vi "ABB Report entered data.vi"(9 "result string in":string, 10 "Efficiency Units":u16(ring) items=["METRIC", "IMPERIAL", "", "", ""], 11 "Efficiency Standard":u16(ring) items=["IEC", "NEMA"]) -> (1 "result string out":string)   [LabVIEW 2017]
uses:
  ABB global.vi
panel:
  out "loads":string[](array[string])
  out "PF&Effy":string[](array[string])
  out "# entries":string[](array[string])
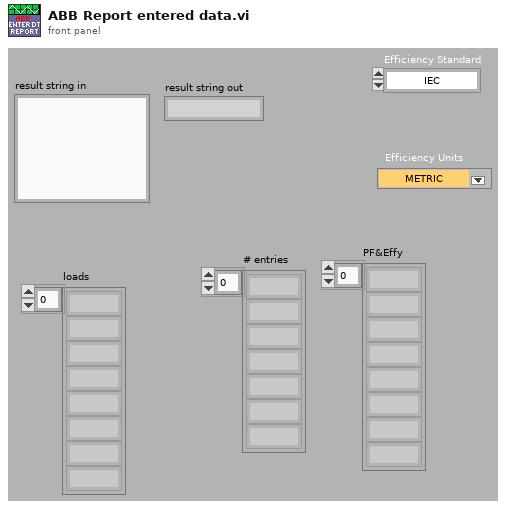
[diagram p1: front panel]
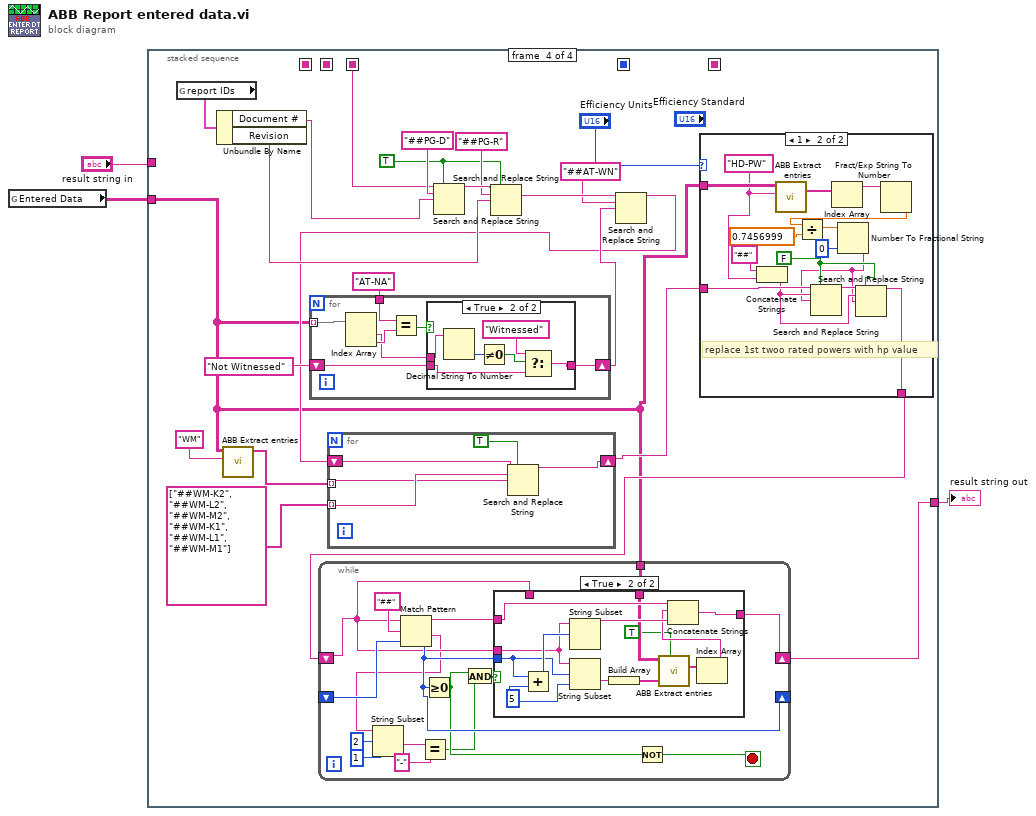
[diagram p0: block diagram]
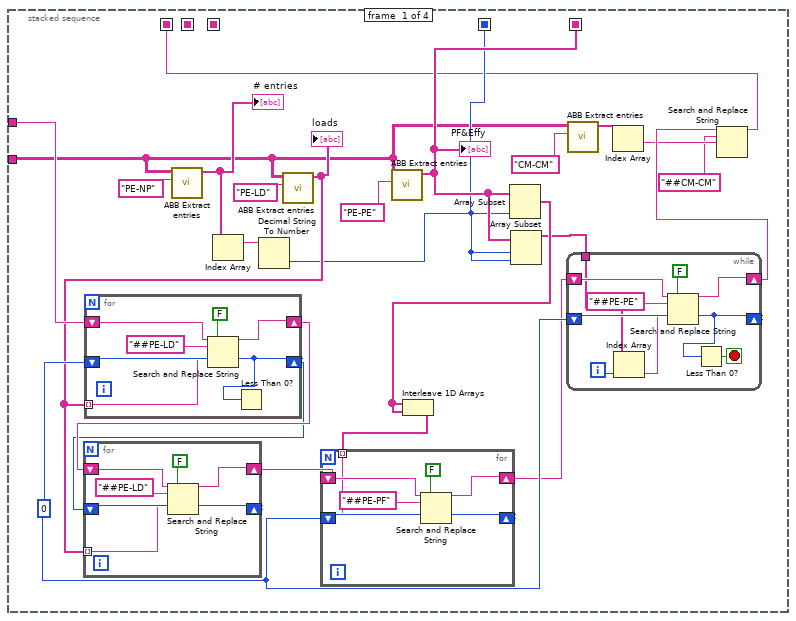
[diagram p2: hidden frame]
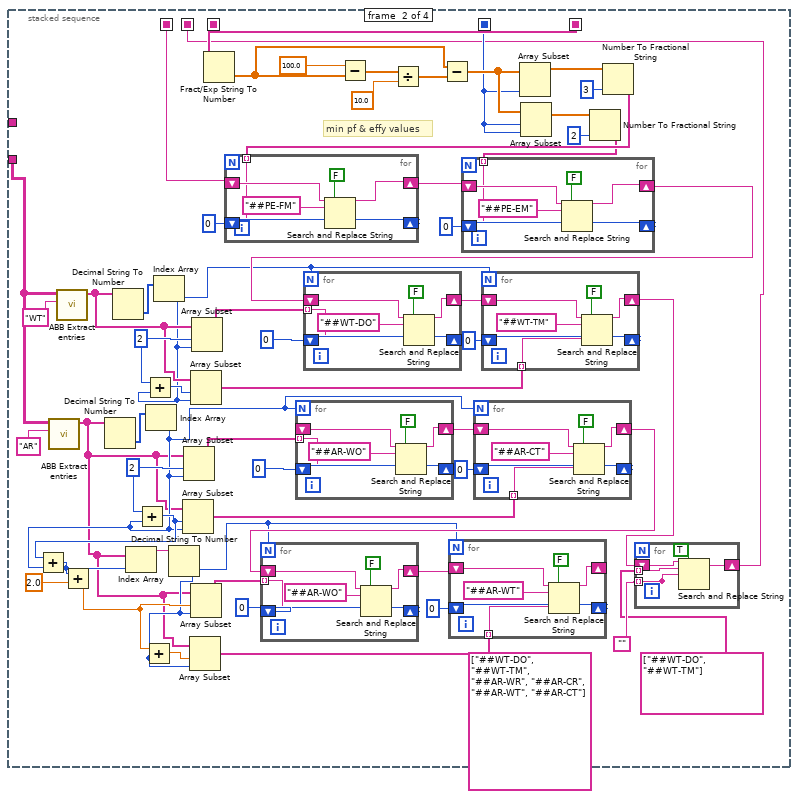
[diagram p3: hidden frame]
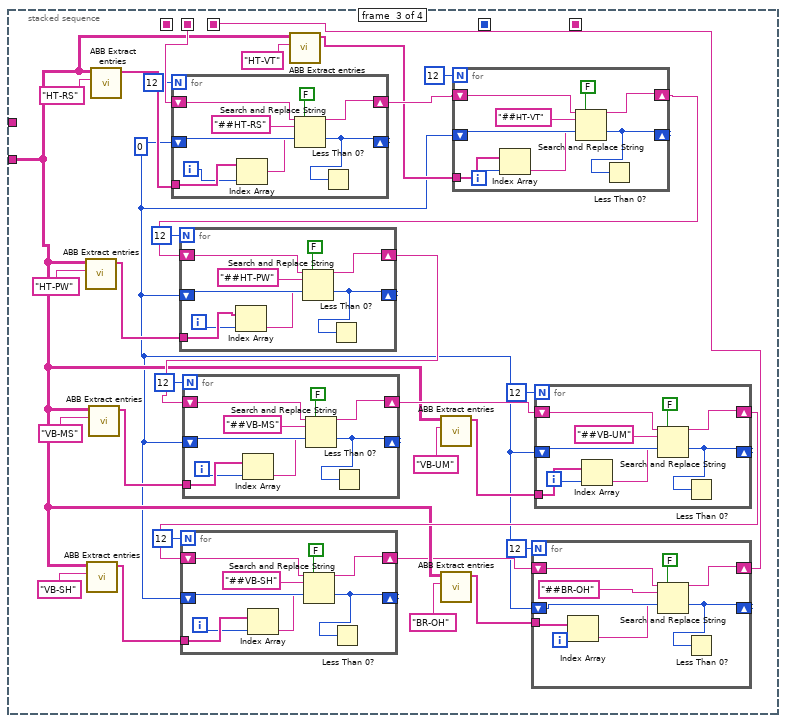
[diagram p4: hidden frame]
diagram:
  n1 = global read "ABB global.vi" "Entered Data"() -> (w1:string[][])
  n2 = stacked-sequence {
    seq-local: [w7 _ _ _] -> [_ w105 _ _]
    seq-local: [w12 _ _ _] -> [_ w116 _ _]
    seq-local: [w11 _ _ _] -> [_ w109 _ _]
    seq-local: [_ w61 _ _] -> [_ _ w206 _]
    seq-local: [_ _ w187 _] -> [_ _ _ w281]
    tunnel: [_ _ _ w280] -> w3
    tunnel: "result string in" -> [w20 _ _ _]
    tunnel: w1 -> [w9 w80 w189 w273]
    frame #0 {
      w21 = 0 ("offset past replacement")
      n3 = call "ABB Extract entries.vi"("Entry ID"="PE-NP" ("element"), "Entry table in"=w9) -> ("Selected Entries"=w24:string[])  [unwired: 9 in]
      "# entries" <- w24
      n4 = Index Array(array=w24) -> (element=w23:string)  [unwired: 1 in]
      n5 = Decimal String To Number(string=w23) -> (number=w11:i32)  [unwired: 2 in, 1 out]
      n6 = call "ABB Extract entries.vi"("Entry ID"="PE-LD" ("element"), "Entry table in"=w9) -> ("Selected Entries"=w17:string[])  [unwired: 9 in]
      "loads" <- w17
      n7 = for {
        shift-right: [w46] -> w19
        shift-left: w20 -> [w48]
        tunnel: w17 -> [w42] mode=indexing
        shift-right: [w43] -> w18
        shift-left: w21 -> [w45]
        n8 = Search and Replace String(replace all?=FALSE ("replace all? (F)"), input string=w48, search string="##PE-LD", replace string=w42, offset=w45) -> (result string=w46:string, offset past replacement=w43:i32)  [unwired: 3 in, 2 out]
        n9 = Less Than 0?(x=w43) -> ()  [unwired: 1 out]
      }
      n10 = for {
        shift-right: [w39] -> w22
        shift-left: w19 -> [w41]
        tunnel: w17 -> [w35] mode=indexing
        shift-right: [w36] -> _
        shift-left: w18 -> [w38]
        n11 = Search and Replace String(replace all?=FALSE ("replace all? (F)"), input string=w41, search string="##PE-LD", replace string=w35, offset=w38) -> (result string=w39:string, offset past replacement=w36:i32)  [unwired: 3 in, 2 out]
      }
      n12 = call "ABB Extract entries.vi"("Entry ID"="PE-PE", "Entry table in"=w9) -> ("Selected Entries"=w12:string[])  [unwired: 9 in]
      "PF&Effy" <- w12
      n13 = Array Subset(array=w12, length=w11) -> (w14:string[])  [unwired: 1 in]
      n14 = Interleave 1D Arrays(w14, w14) -> (w15:string[])
      n15 = for {
        shift-right: [w32] -> w16
        shift-left: w22 -> [w34]
        shift-right: [w29] -> _
        shift-left: w21 -> [w31]
        tunnel: w15 -> [w28] mode=indexing
        n16 = Search and Replace String(replace all?=FALSE ("replace all? (F)"), input string=w34, search string="##PE-PF", replace string=w28, offset=w31) -> (result string=w32:string, offset past replacement=w29:i32)  [unwired: 3 in, 2 out]
      }
      n17 = Array Subset(array=w12, index=w11, length=w11) -> (w13:string[])
      n18 = while {
        shift-right: [w56] -> w6
        shift-left: w16 -> [w58]
        shift-right: [w52] -> _
        shift-left: w21 -> [w55]
        tunnel: w13 -> [w49]
        i -> [w51]
        stop <- w53 stop-if-true
        n19 = Index Array(array=w49, index=w51) -> (element=w50:string)
        n20 = Search and Replace String(replace all?=FALSE ("replace all? (F)"), input string=w58, search string="##PE-PE", replace string=w50, offset=w55) -> (result string=w56:string, offset past replacement=w52:i32)  [unwired: 3 in, 2 out]
        n21 = Less Than 0?(x=w52) -> (x < 0?=w53:bool)
      }
      n22 = call "ABB Extract entries.vi"("Entry ID"="CM-CM", "Entry table in"=w9) -> ("Selected Entries"=w8:string[])  [unwired: 9 in]
      n23 = Index Array(array=w8) -> (element=w5:string)  [unwired: 1 in]
      n24 = Search and Replace String(input string=w6, search string="##CM-CM", replace string=w5) -> (result string=w7:string)  [unwired: 5 in, 3 out]
    }
    frame #1 {
      (unwired) string[] ["##WT-DO", "##WT-TM", "##AR-WR", "##AR-CR", "##AR-WT", "##AR-CT"]
      w84 = 2 ("index")
      w93 = 2 ("index")
      # "min pf & effy values"
      n25 = call "ABB Extract entries.vi"("Entry ID"="AR", "Entry table in"=w80) -> ("Selected Entries"=w63:string[])  [unwired: 9 in]
      n26 = call "ABB Extract entries.vi"("Entry ID"="WT", "Entry table in"=w80) -> ("Selected Entries"=w89:string[])  [unwired: 9 in]
      n27 = Decimal String To Number(string=w63) -> (number=w82:i32[])  [unwired: 2 in, 1 out]
      n28 = Decimal String To Number(string=w89) -> (number=w95:i32[])  [unwired: 2 in, 1 out]
      n29 = Index Array(array=w82) -> (element=w66:i32)  [unwired: 1 in]
      n30 = Add(x=w84, y=w66) -> (x+y=w71:i32)
      n31 = Add(x=w71, y=w66) -> (x+y=w70:i32)
      n32 = Add(x=w70, y=2.0) -> (x+y=w68:dbl)
      n33 = Index Array(array=w63, index=w70) -> (element=w67:string)
      n34 = Index Array(array=w95) -> (element=w64:i32)  [unwired: 1 in]
      n35 = Add(x=w93, y=w64) -> (x+y=w92:i32)
      n36 = Decimal String To Number(string=w67) -> (number=w65:i32)  [unwired: 2 in, 1 out]
      n37 = Add(x=w68, y=w65) -> (x+y=w76:dbl)
      n38 = Array Subset(array=w63, index=w71, length=w66) -> (w87:string[])
      n39 = Array Subset(array=w63, index=w84, length=w66) -> (w83:string[])
      n40 = Array Subset(array=w63, index=w76, length=w65) -> (w73:string[])
      n41 = Array Subset(array=w89, index=w92, length=w64) -> (w88:string[])
      n42 = Array Subset(array=w63, index=w68, length=w65) -> (w77:string[])
      n43 = Array Subset(array=w89, index=w93, length=w64) -> (w94:string[])
      n44 = Fract/Exp String To Number(string=w116) -> (number=w112:dbl[])  [unwired: 3 in, 1 out]
      n45 = for {
        N: w66 -> [_]
        shift-right: [w147] -> w85
        shift-left: _ -> [w149]
        shift-right: [w144] -> _
        shift-left: 0 ("offset past replacement") -> [w146]
        tunnel: w83 -> [w143] mode=indexing
        n46 = Search and Replace String(replace all?=FALSE ("replace all? (F)"), input string=w149, search string="##AR-WO", replace string=w143, offset=w146) -> (result string=w147:string, offset past replacement=w144:i32)  [unwired: 3 in, 2 out]
      }
      n47 = Subtract(x=100.0, y=w112) -> (x-y=w114:dbl[])
      n48 = Divide(x=w114, y=10.0) -> (x/y=w111:dbl[])
      n49 = Subtract(x=w112, y=w111) -> (x-y=w110:dbl[])
      n50 = for {
        N: w66 -> [_]
        shift-right: [w140] -> w72
        shift-left: w85 -> [w142]
        shift-right: [w137] -> _
        shift-left: 0 ("offset past replacement") -> [w139]
        tunnel: w87 -> [w136] mode=indexing
        n51 = Search and Replace String(replace all?=FALSE ("replace all? (F)"), input string=w142, search string="##AR-CT", replace string=w136, offset=w139) -> (result string=w140:string, offset past replacement=w137:i32)  [unwired: 3 in, 2 out]
      }
      n52 = for {
        N: w65 -> [_]
        shift-right: [w133] -> w75
        shift-left: w72 -> [w135]
        shift-right: [w130] -> _
        shift-left: 0 ("offset past replacement") -> [w132]
        tunnel: w77 -> [w129] mode=indexing
        n53 = Search and Replace String(replace all?=FALSE ("replace all? (F)"), input string=w135, search string="##AR-WO", replace string=w129, offset=w132) -> (result string=w133:string, offset past replacement=w130:i32)  [unwired: 3 in, 2 out]
      }
      n54 = for {
        N: w65 -> [_]
        shift-right: [w126] -> _
        shift-left: w75 -> [w128]
        shift-right: [w123] -> _
        shift-left: 0 ("offset past replacement") -> [w125]
        tunnel: w73 -> [w122] mode=indexing
        n55 = Search and Replace String(replace all?=FALSE ("replace all? (F)"), input string=w128, search string="##AR-WT", replace string=w122, offset=w125) -> (result string=w126:string, offset past replacement=w123:i32)  [unwired: 3 in, 2 out]
      }
      n56 = Array Subset(array=w110, length=w109) -> (w108:dbl[])  [unwired: 1 in]
      n57 = Array Subset(array=w110, index=w109, length=w109) -> (w102:dbl[])
      n58 = Number To Fractional String(number=w102, precision (6)=i16 2) -> (F-format string=w100:string[])  [unwired: 2 in]
      n59 = Number To Fractional String(number=w108, precision (6)=i16 3) -> (F-format string=w106:string[])  [unwired: 2 in]
      n60 = for {
        shift-right: [w175] -> w103
        shift-left: w105 -> [w177]
        shift-right: [w172] -> _
        shift-left: 0 ("offset past replacement") -> [w174]
        tunnel: w106 -> [w171] mode=indexing
        n61 = Search and Replace String(replace all?=FALSE ("replace all? (F)"), input string=w177, search string="##PE-FM", replace string=w171, offset=w174) -> (result string=w175:string, offset past replacement=w172:i32)  [unwired: 3 in, 2 out]
      }
      n62 = for {
        shift-right: [w168] -> w98
        shift-left: w103 -> [w170]
        shift-right: [w165] -> _
        shift-left: 0 ("offset past replacement") -> [w167]
        tunnel: w100 -> [w164] mode=indexing
        n63 = Search and Replace String(replace all?=FALSE ("replace all? (F)"), input string=w170, search string="##PE-EM", replace string=w164, offset=w167) -> (result string=w168:string, offset past replacement=w165:i32)  [unwired: 3 in, 2 out]
      }
      n64 = for {
        N: w64 -> [_]
        shift-right: [w161] -> w91
        shift-left: w98 -> [w163]
        shift-right: [w158] -> _
        shift-left: 0 ("offset past replacement") -> [w160]
        tunnel: w94 -> [w157] mode=indexing
        n65 = Search and Replace String(replace all?=FALSE ("replace all? (F)"), input string=w163, search string="##WT-DO", replace string=w157, offset=w160) -> (result string=w161:string, offset past replacement=w158:i32)  [unwired: 3 in, 2 out]
      }
      n66 = for {
        N: w64 -> [_]
        shift-right: [w154] -> w60
        shift-left: w91 -> [w156]
        shift-right: [w151] -> _
        shift-left: 0 ("offset past replacement") -> [w153]
        tunnel: w88 -> [w150] mode=indexing
        n67 = Search and Replace String(replace all?=FALSE ("replace all? (F)"), input string=w156, search string="##WT-TM", replace string=w150, offset=w153) -> (result string=w154:string, offset past replacement=w151:i32)  [unwired: 3 in, 2 out]
      }
      n68 = for {
        shift-right: [w120] -> w61
        shift-left: w60 -> [w121]
        tunnel: string[] ["##WT-DO", "##WT-TM"] -> [w118] mode=indexing
        tunnel: "" -> [w117]
        tunnel: [w117] -> _ mode=indexing
        n69 = Search and Replace String(replace all?=TRUE ("replace all? (F)"), input string=w121, search string=w118, replace string=w117) -> (result string=w120:string)  [unwired: 4 in, 3 out]
      }
    }
    frame #2 {
      w186 = 0 ("offset past replacement")
      n70 = call "ABB Extract entries.vi"("Entry ID"="HT-PW", "Entry table in"=w189) -> ("Selected Entries"=w200:string[])  [unwired: 9 in]
      n71 = call "ABB Extract entries.vi"("Entry ID"="VB-SH", "Entry table in"=w189) -> ("Selected Entries"=w197:string[])  [unwired: 9 in]
      n72 = call "ABB Extract entries.vi"("Entry ID"="VB-MS", "Entry table in"=w189) -> ("Selected Entries"=w199:string[])  [unwired: 9 in]
      n73 = call "ABB Extract entries.vi"("Entry ID"="HT-RS", "Entry table in"=w189) -> ("Selected Entries"=w207:string[])  [unwired: 9 in]
      n74 = for {
        N: 12 -> [_]
        shift-right: [w269] -> w205
        shift-left: w206 -> [w271]
        tunnel: w207 -> [w265]
        shift-right: [w266] -> _
        shift-left: w186 -> [w268]
        i -> [w264]
        n75 = Index Array(array=w265, index=w264) -> (element=w263:string)
        n76 = Search and Replace String(replace all?=FALSE ("replace all? (F)"), input string=w271, search string="##HT-RS", replace string=w263, offset=w268) -> (result string=w269:string, offset past replacement=w266:i32)  [unwired: 3 in, 2 out]
        n77 = Less Than 0?(x=w266) -> ()  [unwired: 1 out]
      }
      n78 = call "ABB Extract entries.vi"("Entry ID"="HT-VT", "Entry table in"=w189) -> ("Selected Entries"=w202:string[])  [unwired: 9 in]
      n79 = call "ABB Extract entries.vi"("Entry ID"="VB-UM", "Entry table in"=w189) -> ("Selected Entries"=w198:string[])  [unwired: 9 in]
      n80 = call "ABB Extract entries.vi"("Entry ID"="BR-OH", "Entry table in"=w189) -> ("Selected Entries"=w185:string[])  [unwired: 9 in]
      n81 = for {
        N: 12 -> [_]
        shift-right: [w260] -> w204
        shift-left: w205 -> [w262]
        tunnel: w202 -> [w256]
        shift-right: [w257] -> _
        shift-left: w186 -> [w259]
        i -> [w254]
        n82 = Index Array(array=w256, index=w254) -> (element=w255:string)
        n83 = Search and Replace String(replace all?=FALSE ("replace all? (F)"), input string=w262, search string="##HT-VT", replace string=w255, offset=w259) -> (result string=w260:string, offset past replacement=w257:i32)  [unwired: 3 in, 2 out]
        n84 = Less Than 0?(x=w257) -> ()  [unwired: 1 out]
      }
      n85 = for {
        N: 12 -> [_]
        shift-right: [w251] -> w194
        shift-left: w204 -> [w253]
        tunnel: w200 -> [w247]
        shift-right: [w248] -> _
        shift-left: w186 -> [w250]
        i -> [w246]
        n86 = Index Array(array=w247, index=w246) -> (element=w245:string)
        n87 = Search and Replace String(replace all?=FALSE ("replace all? (F)"), input string=w253, search string="##HT-PW", replace string=w245, offset=w250) -> (result string=w251:string, offset past replacement=w248:i32)  [unwired: 3 in, 2 out]
        n88 = Less Than 0?(x=w248) -> ()  [unwired: 1 out]
      }
      n89 = for {
        N: 12 -> [_]
        shift-right: [w242] -> w195
        shift-left: w194 -> [w244]
        tunnel: w199 -> [w238]
        shift-right: [w239] -> _
        shift-left: w186 -> [w241]
        i -> [w236]
        n90 = Index Array(array=w238, index=w236) -> (element=w237:string)
        n91 = Search and Replace String(replace all?=FALSE ("replace all? (F)"), input string=w244, search string="##VB-MS", replace string=w237, offset=w241) -> (result string=w242:string, offset past replacement=w239:i32)  [unwired: 3 in, 2 out]
        n92 = Less Than 0?(x=w239) -> ()  [unwired: 1 out]
      }
      n93 = for {
        N: 12 -> [_]
        shift-right: [w233] -> w193
        shift-left: w195 -> [w235]
        tunnel: w198 -> [w229]
        shift-right: [w230] -> _
        shift-left: w186 -> [w232]
        i -> [w227]
        n94 = Index Array(array=w229, index=w227) -> (element=w228:string)
        n95 = Search and Replace String(replace all?=FALSE ("replace all? (F)"), input string=w235, search string="##VB-UM", replace string=w228, offset=w232) -> (result string=w233:string, offset past replacement=w230:i32)  [unwired: 3 in, 2 out]
        n96 = Less Than 0?(x=w230) -> ()  [unwired: 1 out]
      }
      n97 = for {
        N: 12 -> [_]
        shift-right: [w224] -> w188
        shift-left: w193 -> [w226]
        tunnel: w197 -> [w220]
        shift-right: [w221] -> _
        shift-left: w186 -> [w223]
        i -> [w218]
        n98 = Index Array(array=w220, index=w218) -> (element=w219:string)
        n99 = Search and Replace String(replace all?=FALSE ("replace all? (F)"), input string=w226, search string="##VB-SH", replace string=w219, offset=w223) -> (result string=w224:string, offset past replacement=w221:i32)  [unwired: 3 in, 2 out]
        n100 = Less Than 0?(x=w221) -> ()  [unwired: 1 out]
      }
      n101 = for {
        N: 12 -> [_]
        shift-right: [w215] -> w187
        shift-left: w188 -> [w217]
        tunnel: w185 -> [w211]
        shift-right: [w212] -> _
        shift-left: w186 -> [w214]
        i -> [w210]
        n102 = Index Array(array=w211, index=w210) -> (element=w209:string)
        n103 = Search and Replace String(replace all?=FALSE ("replace all? (F)"), input string=w217, search string="##BR-OH", replace string=w209, offset=w214) -> (result string=w215:string, offset past replacement=w212:i32)  [unwired: 3 in, 2 out]
        n104 = Less Than 0?(x=w212) -> ()  [unwired: 1 out]
      }
    }
    frame #3 {
      w290 = TRUE ("replace all? (F)")
      n105 = global read "ABB global.vi" "report IDs"() -> (w282:cluster{"Document #":string, "Revision":string})
      n106 = Unbundle By Name(w282) -> ("Document #"=w283:string, "Revision"=w284:string)
      n107 = call "ABB Extract entries.vi"("Entry ID"="WM", "Entry table in"=w273) -> ("Selected Entries"=w278:string[])  [unwired: 9 in]
      n108 = for {
        tunnel: w273 -> [w321] mode=indexing
        tunnel: "AT-NA" -> [w319]
        shift-right: [w316] -> w285
        shift-left: "Not Witnessed" -> [w317]
        n109 = Index Array(array=w321) -> (element #1=w315:string, element #2=w320:string)  [unwired: 2 in]
        n110 = Equal?(x=w319, y=w320) -> (x = y?=w318:bool)
        n111 = case shown="True" w318 {
          tunnel: w317 -> [w322 w327]
          tunnel: [w322 w326] -> w316
          tunnel: w315 -> [_ w328]
          frame False {
          }
          frame True {
            n112 = Decimal String To Number(string=w328) -> (number=w325:i32)  [unwired: 2 in, 1 out]
            n113 = Not Equal To 0?(x=w325) -> (x != 0?=w324:bool)
            n114 = Select(t="Witnessed", s=w324, f=w327) -> (s? t:f=w326:string)
          }
        }
      }
      n115 = Search and Replace String(replace all?=w290, input string=w281, search string="##PG-D", replace string=w283) -> (result string=w292:string)  [unwired: 4 in, 3 out]
      n116 = Search and Replace String(replace all?=w290, input string=w292, search string="##PG-R", replace string=w284) -> (result string=w289:string)  [unwired: 4 in, 3 out]
      n117 = Search and Replace String(input string=w289, search string="##AT-WN" ("substring (\"\")"), replace string=w285) -> (result string=w276:string)  [unwired: 5 in, 3 out]
      n118 = for {
        shift-right: [w313] -> w275
        shift-left: w276 -> [w314]
        tunnel: w278 -> [w310] mode=indexing
        tunnel: string[] ["##WM-K2", "##WM-L2", "##WM-M2", "##WM-K1", "##WM-L1", "##WM-M1"] -> [w312] mode=indexing
        n119 = Search and Replace String(replace all?=TRUE ("replace all? (F)"), input string=w314, search string=w312, replace string=w310) -> (result string=w313:string)  [unwired: 4 in, 3 out]
      }
      n120 = case shown="1" "Efficiency Units" {
        tunnel: w273 -> [_ w309]
        tunnel: [w294 w298] -> w274
        tunnel: w275 -> [w294 w303]
        frame 0, Default {
        }
        frame 1 {
          w297 = FALSE ("replace all? (F)")
          w302 = "HD-PW" ("Entry ID")
          # "replace 1st twoo rated powers with hp value"
          n121 = Concatenate Strings("##" ("string"), w302) -> (w296:string)
          n122 = call "ABB Extract entries.vi"("Entry ID"=w302, "Entry table in"=w309) -> ("Selected Entries"=w308:string[])  [unwired: 9 in]
          n123 = Index Array(array=w308) -> (element=w307:string)  [unwired: 1 in]
          n124 = Fract/Exp String To Number(string=w307) -> (number=w306:dbl)  [unwired: 3 in, 1 out]
          n125 = Divide(x=w306, y=0.7456999) -> (x/y=w304:dbl)
          n126 = Number To Fractional String(number=w304, precision (6)=i16 0) -> (F-format string=w295:string)  [unwired: 2 in]
          n127 = Search and Replace String(replace all?=w297, input string=w303, search string=w296, replace string=w295) -> (result string=w299:string)  [unwired: 4 in, 3 out]
          n128 = Search and Replace String(replace all?=w297, input string=w299, search string=w296, replace string=w295) -> (result string=w298:string)  [unwired: 4 in, 3 out]
        }
      }
      n129 = while {
        shift-right: [w342] -> w280
        shift-left: w274 -> [w338]
        shift-right: [w340] -> _
        shift-left: _ -> [w339]
        tunnel: w273 -> [w341]
        stop <- w332 stop-if-true
        n130 = Match Pattern(string=w338, regular expression="##", offset (0)=w339) -> (before substring=w343:string, after substring=w337:string, offset past match=w340:i32)  [unwired: 1 out]
        n131 = String Subset(string=w337, offset (0)=2, length (rest)=1 ("length (rest)")) -> (substring=w334:string)
        n132 = Equal?(x=w334, y="-") -> (x = y?=w329:bool)
        n133 = Greater Or Equal To 0?(x=w340) -> (x >= 0?=w330:bool)
        n134 = And(x=w330, y=w329) -> (x .and. y?=w331:bool)
        n135 = case shown="True" w331 {
          tunnel: w343 -> [_ w358]
          tunnel: [w345 w357] -> w342
          tunnel: w341 -> [_ w353]
          tunnel: w340 -> [_ w350]
          tunnel: w338 -> [w345 _]
          tunnel: w338 -> [_ w347]
          frame False {
          }
          frame True {
            w354 = 5 ("y")
            n136 = Add(x=w350, y=w354) -> (x+y=w356:i32)
            n137 = String Subset(string=w347, offset (0)=w356) -> (substring=w355:string)  [unwired: 1 in]
            n138 = String Subset(string=w347, offset (0)=w350, length (rest)=w354) -> (substring=w349:string)
            n139 = Build Array(w349) -> (w348:string[])
            n140 = call "ABB Extract entries.vi"("Pulldown text"=TRUE, "Entry IDs"=w348, "Entry table in"=w353) -> ("Selected Entries"=w352:string[])  [unwired: 8 in]
            n141 = Index Array(array=w352) -> (element=w351:string)  [unwired: 1 in]
            n142 = Concatenate Strings(w358, w351, w355) -> (w357:string)
          }
        }
        n143 = Not(x=w330) -> (.not. x?=w332:bool)
      }
    }
  }
  "result string out" <- w3
